vi "剖面多参数上传.vi"(11 "错误输入（无错误）":errorcluster) -> (15 "error out":errorcluster)   [LabVIEW 2016, in "数据传输系统.lvlib"]
uses:
  <vilib>/Utility/config.llb/Write Key (String).vi
  <vilib>/Utility/config.llb/NI_LVConfig.lvlib
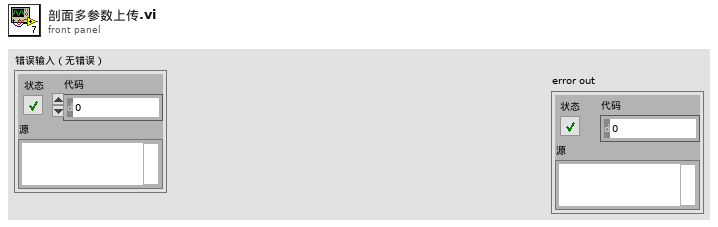
[diagram p1: front panel]
types:
  T1 = typedef "NI_LVConfig.lvlib/Config Data RefNum.ctl" = refnum<k1>
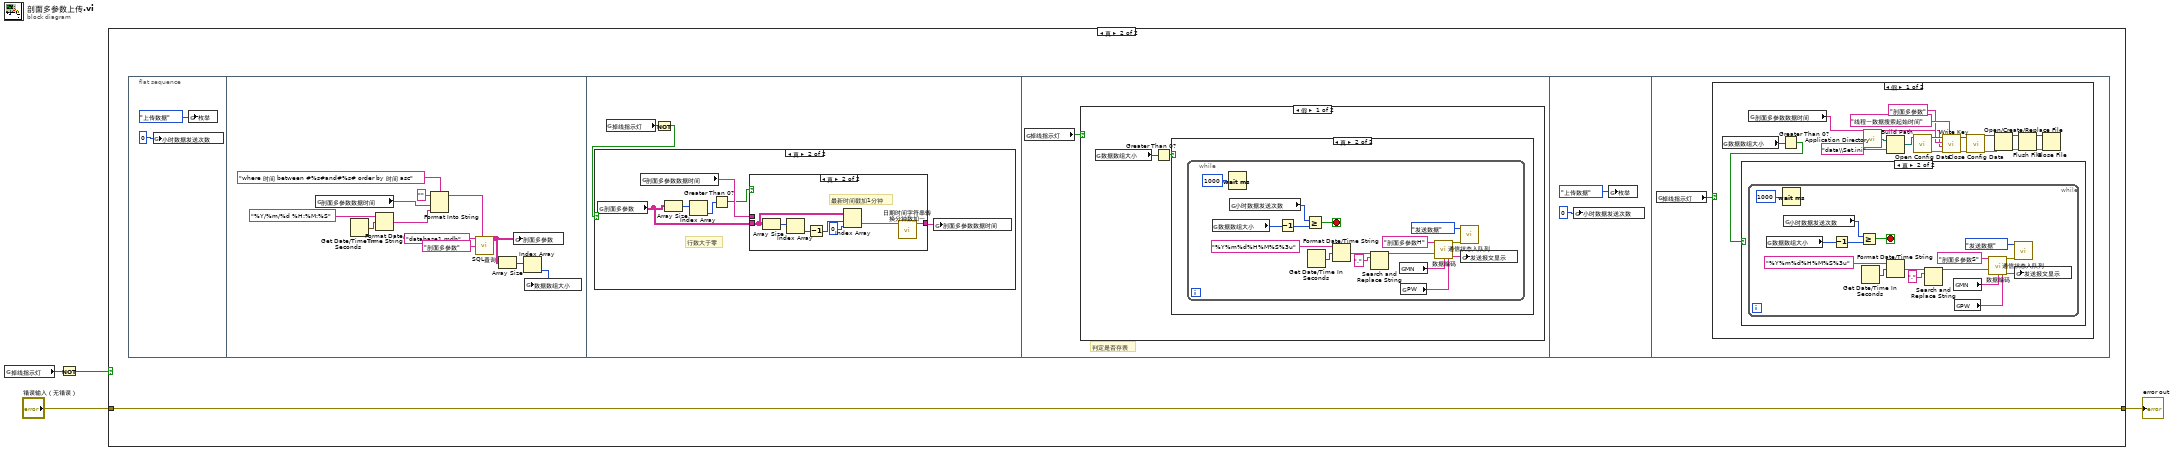
[diagram p0: block diagram]
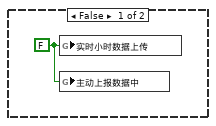
[diagram p2: hidden frame]
diagram:
  n1 = global read "全局 数据发送重叠.vi" "掉线指示灯"() -> (w4:bool)
  n2 = Not(x=w4) -> (.not. x?=w1:bool)
  n3 = case shown="真" w1 {
    tunnel: [_ w6] -> w3
    tunnel: "错误输入（无错误）" -> [_ w6]
    frame False {
      w5 = FALSE ("小时数据上传")
      n4 = global write "全局1.vi" "实时小时数据上传"(w5) -> ()
      n5 = global write "全局 数据发送重叠.vi" "主动上报数据中"(w5) -> ()
    }
    frame True {
      n6 = flat-sequence {
        frame #0 {
          n7 = global write "全局 小时数据发送次数.vi" "小时数据发送次数"(0 ("小时数据发送次数")) -> ()
          n8 = global write "全局1.vi" "枚举"(enum16{"返回请求应答", "上传数据", "返回执行结果"}."上传数据" ("枚举")) -> ()
        }
        frame #1 {
          n9 = global read "全局 水样时间.vi" "剖面多参数数据时间"() -> (w14:string)
          n10 = Get Date/Time In Seconds() -> (seconds since 1Jan1904=w18:timestamp)
          n11 = Format Date/Time String(time format string (%c)="%Y/%m/%d %H:%M:%S" ("时间格式字符串(%c)"), seconds (now)=w18) -> (date/time string=w13:string)  [unwired: 1 in]
          n12 = Format Into String(format string="where 时间 between #%s#and#%s# order by 时间 asc" ("condition"), initial string="" ("初始字符串"), w14, w13) -> (resulting string=w12:string)  [unwired: 1 in, 1 out]
          n13 = call "SQL查询.vi"("condition"=w12, "table输入"="剖面多参数", "database"="database1.mdb") -> ("data"=w11:string[][])  [unwired: 6 in, 2 out]
          n14 = Array Size(array=w11) -> (size(s)=w10:i32[])
          n15 = global write "全局 所有参数.vi" "剖面多参数"(w11) -> ()
          n16 = Index Array(array=w10) -> (element=w9:i32)  [unwired: 1 in]
          n17 = global write "全局 数据数组大小.vi" "数据数组大小"(w9) -> ()
        }
        frame #2 {
          n18 = global read "全局 数据发送重叠.vi" "掉线指示灯"() -> (w22:bool)
          n19 = Not(x=w22) -> (.not. x?=w21:bool)
          n20 = case shown="真" w21 {
            frame False {
            }
            frame True {
              # "行数大于零"
              n21 = global read "全局 所有参数.vi" "剖面多参数"() -> (w27:string[][])
              n22 = global read "全局 水样时间.vi" "剖面多参数数据时间"() -> (w28:string)
              n23 = Array Size(array=w27) -> (size(s)=w24:i32[])
              n24 = Index Array(array=w24) -> (element=w25:i32)  [unwired: 1 in]
              n25 = Greater Than 0?(x=w25) -> (x > 0?=w26:bool)
              n26 = case shown="真" w26 {
                tunnel: w27 -> [_ w33]
                tunnel: [w29 w30] -> w23
                tunnel: w28 -> [w29 _]
                frame False {
                }
                frame True {
                  # "最新时间戳加1分钟"
                  n27 = Array Size(array=w33) -> (size(s)=w35:i32[])
                  n28 = Index Array(array=w35) -> (element=w34:i32)  [unwired: 1 in]
                  n29 = Decrement(x=w34) -> (x-1=w32:i32)
                  n30 = Index Array(array=w33, index (row)=w32, index (col)=0 ("禁用的索引 (列)")) -> (element=w36:string)
                  n31 = call "日期时间字符串转换分钟数加一.vi"("data[0]"=w36) -> ("日期/时间字符串"=w30:string)  [unwired: 10 in]
                }
              }
              n32 = global write "全局 水样时间.vi" "剖面多参数数据时间"(w23) -> ()
            }
          }
        }
        frame #3 {
          # "判定是否存表"
          n33 = global read "全局 数据发送重叠.vi" "掉线指示灯"() -> (w37:bool)
          n34 = case shown="假" w37 {
            frame False {
              n35 = global read "全局 数据数组大小.vi" "数据数组大小"() -> (w38:i32)
              n36 = Greater Than 0?(x=w38) -> (x > 0?=w39:bool)
              n37 = case shown="真" w39 {
                frame False {
                }
                frame True {
                  n38 = while {
                    stop <- w40 stop-if-true
                    n39 = global read "全局 数据数组大小.vi" "数据数组大小"() -> (w42:i32)
                    n40 = Wait (ms)(milliseconds to wait=u32 1000 ("等待时间（毫秒）")) -> ()  [unwired: 1 out]
                    n41 = global read "全局 小时数据发送次数.vi" "小时数据发送次数"() -> (w43:i32)
                    n42 = Decrement(x=w42) -> (x-1=w41:i32)
                    n43 = Greater Or Equal?(x=w43, y=w41) -> (x >= y?=w40:bool)
                    n44 = Get Date/Time In Seconds() -> (seconds since 1Jan1904=w53:timestamp)
                    n45 = Format Date/Time String(time format string (%c)="%Y%m%d%H%M%S%3u" ("时间格式字符串(%c)"), seconds (now)=w53) -> (date/time string=w52:string)  [unwired: 1 in]
                    n46 = Search and Replace String(input string=w52, search string="." ("搜索字符串")) -> (result string=w50:string)  [unwired: 6 in, 3 out]
                    n47 = global read "断电保存全局.vi" "MN"() -> (w47:string)
                    n48 = global read "断电保存全局.vi" "PW"() -> (w46:string)
                    n49 = call "数据编码.vi"("table输入"="剖面多参数H" ("新元素/子数组"), "QN"=w50, "MN"=w47, "PW"=w46) -> ("错误常量"=w45:errorcluster, "通讯包字符串"=w49:string)  [unwired: 10 in]
                    n50 = call "通信状态入队列.vi"("错误输入（无错误）"=w45, "枚举"=enum16{"打开连接", "发送数据", "读取数据", "数据处理", "关闭连接"}."发送数据") -> ()  [unwired: 9 in, 1 out]
                    n51 = global write "全局1.vi" "发送报文显示"(w49) -> ()
                  }
                }
              }
            }
            frame True {
            }
          }
        }
        frame #4 {
          n52 = global write "全局 小时数据发送次数.vi" "小时数据发送次数"(0 ("小时数据发送次数")) -> ()
          n53 = global write "全局1.vi" "枚举"(enum16{"返回请求应答", "上传数据", "返回执行结果"}."上传数据" ("枚举")) -> ()
        }
        frame #5 {
          n54 = global read "全局 数据发送重叠.vi" "掉线指示灯"() -> (w58:bool)
          n55 = case shown="假" w58 {
            frame False {
              n56 = global read "全局 数据数组大小.vi" "数据数组大小"() -> (w76:i32)
              n57 = global read "全局 水样时间.vi" "剖面多参数数据时间"() -> (w59:string)
              n58 = Greater Than 0?(x=w76) -> (x > 0?=w75:bool)
              n59 = case shown="真" w75 {
                frame False {
                }
                frame True {
                  n60 = while {
                    stop <- w77 stop-if-true
                    n61 = global read "全局 数据数组大小.vi" "数据数组大小"() -> (w79:i32)
                    n62 = Wait (ms)(milliseconds to wait=u32 1000 ("等待时间（毫秒）")) -> ()  [unwired: 1 out]
                    n63 = global read "全局 小时数据发送次数.vi" "小时数据发送次数"() -> (w80:i32)
                    n64 = Decrement(x=w79) -> (x-1=w78:i32)
                    n65 = Greater Or Equal?(x=w80, y=w78) -> (x >= y?=w77:bool)
                    n66 = Get Date/Time In Seconds() -> (seconds since 1Jan1904=w90:timestamp)
                    n67 = Format Date/Time String(time format string (%c)="%Y%m%d%H%M%S%3u" ("时间格式字符串(%c)"), seconds (now)=w90) -> (date/time string=w89:string)  [unwired: 1 in]
                    n68 = Search and Replace String(input string=w89, search string="." ("搜索字符串")) -> (result string=w87:string)  [unwired: 6 in, 3 out]
                    n69 = global read "断电保存全局.vi" "MN"() -> (w84:string)
                    n70 = global read "断电保存全局.vi" "PW"() -> (w83:string)
                    n71 = call "数据编码.vi"("table输入"="剖面多参数S" ("新元素/子数组"), "QN"=w87, "MN"=w84, "PW"=w83) -> ("错误常量"=w82:errorcluster, "通讯包字符串"=w86:string)  [unwired: 10 in]
                    n72 = call "通信状态入队列.vi"("错误输入（无错误）"=w82, "枚举"=enum16{"打开连接", "发送数据", "读取数据", "数据处理", "关闭连接"}."发送数据") -> ()  [unwired: 9 in, 1 out]
                    n73 = global write "全局1.vi" "发送报文显示"(w86) -> ()
                  }
                }
              }
              n74 = call <vilib>:"Application Directory.vi"() -> ("Application Directory"=w67:path)
              n75 = Build Path(base path=w67, name or relative path="data\\Set.ini" ("名称或相对路径")) -> (appended path=w69:path)
              n76 = call <vilib>:"Open Config Data.vi"("configuration file path"=w69) -> ("error out"=w71:errorcluster, "refnum"=w70:T1)  [unwired: 8 in, 1 out]
              n77 = call-poly <vilib>:"Write Key.vi"("section"="线程一数据搜索起始时间", "error in (no error)"=w71, "value"=w59, "key"="剖面多参数", "refnum"=w70) -> ("error out"=w73:errorcluster, "refnum out"=w72:T1)  [unwired: 4 in, 1 out]
              n78 = call <vilib>:"Close Config Data.vi"("error in (no error)"=w73, "refnum"=w72) -> ("error out"=w60:errorcluster, "file path"=w61:path)  [unwired: 8 in]
              n79 = Open/Create/Replace File(file path (use dialog)=w61, error in=w60) -> (refnum out=w63:refnum<file>, error out=w62:errorcluster)  [unwired: 4 in, 1 out]
              n80 = Flush File(refnum=w63, error in=w62) -> (refnum out=w64:refnum<file>, error out=w65:errorcluster)
              n81 = Close File(refnum=w64, error in=w65) -> ()  [unwired: 2 out]
            }
            frame True {
            }
          }
        }
      }
    }
  }
  "error out" <- w3
